vi "Main.vi"() -> ()   [LabVIEW 2018]
doc: "This template is for the Queued Message Handler design pattern.\n\nThe Event Handling Loop generates messages based on user interface actions.\n\nThe Message Handling Loop processes messages generated by the Event Handling Loop, or by other messages. The messages are string values, so new messages can be added easily to the Message Cases case structure in the Message Handling Loop. Each message cluster can also provide an optional value for Message Data, which is a variant that can be converted to whatever message-specific data is required."
uses:
  Type Defs/SR Cluster.ctl
  Type Defs/SR Status.ctl
  Type Defs/Filter Cluster.ctl
  Type Defs/Sorting Methods.ctl
  Support/Message Queue/Enqueue Message (Single).vi
  Support/Message Queue/Message Queue.lvlib
  Support/User Events/User Events.lvlib
panel:
  in  "Remove SR":bool
  in  "Legend":cluster{"Color Box":u32, "String":string}[][](array[cluster])=[[{"Color Box"=16750899, "String"="In Work (Answer Today)"}, {"Color Box"=6737151, "String"="In Collab"}, {"Color Box"=16735833, "String"="Past Due"}], [{"Color Box"=14417800, "String"="In Work"}, {"Color Box"=4713287, "String"="Potentially Resolved"}, {"Color Box"=16580608, "String"="Passed Off"}], [{"Color Box"=3342591, "String"="In Collab (Answer Today)"}, {"Color Box"=9746580, "String"="Resolved"}, {"Color Box"=0, "String"="Other"}]]
  out "Message":string
  out "Labels":string="          SR#          SR Status                          Name                                 Summary                                                                         Last Updated      SR Type                 Service Level        Open      Create Date"
  in  "Sorting":T1
  in  "Filter Cluster":T2={"Show Resolved"=TRUE, "Show Potentially Resolved"=TRUE, "Show Passoffs"=TRUE, "Show In Collab"=TRUE}
  in  "Add SR":bool
  out "SR Display List":T3[](array[typedef]) {"Creation Date" format="%<%x>T"; "Last Updated" format="%<%x>T"; "Days Open" format="%#.1f"}
  in  "Refresh SRs":bool
  in  "Exit":bool
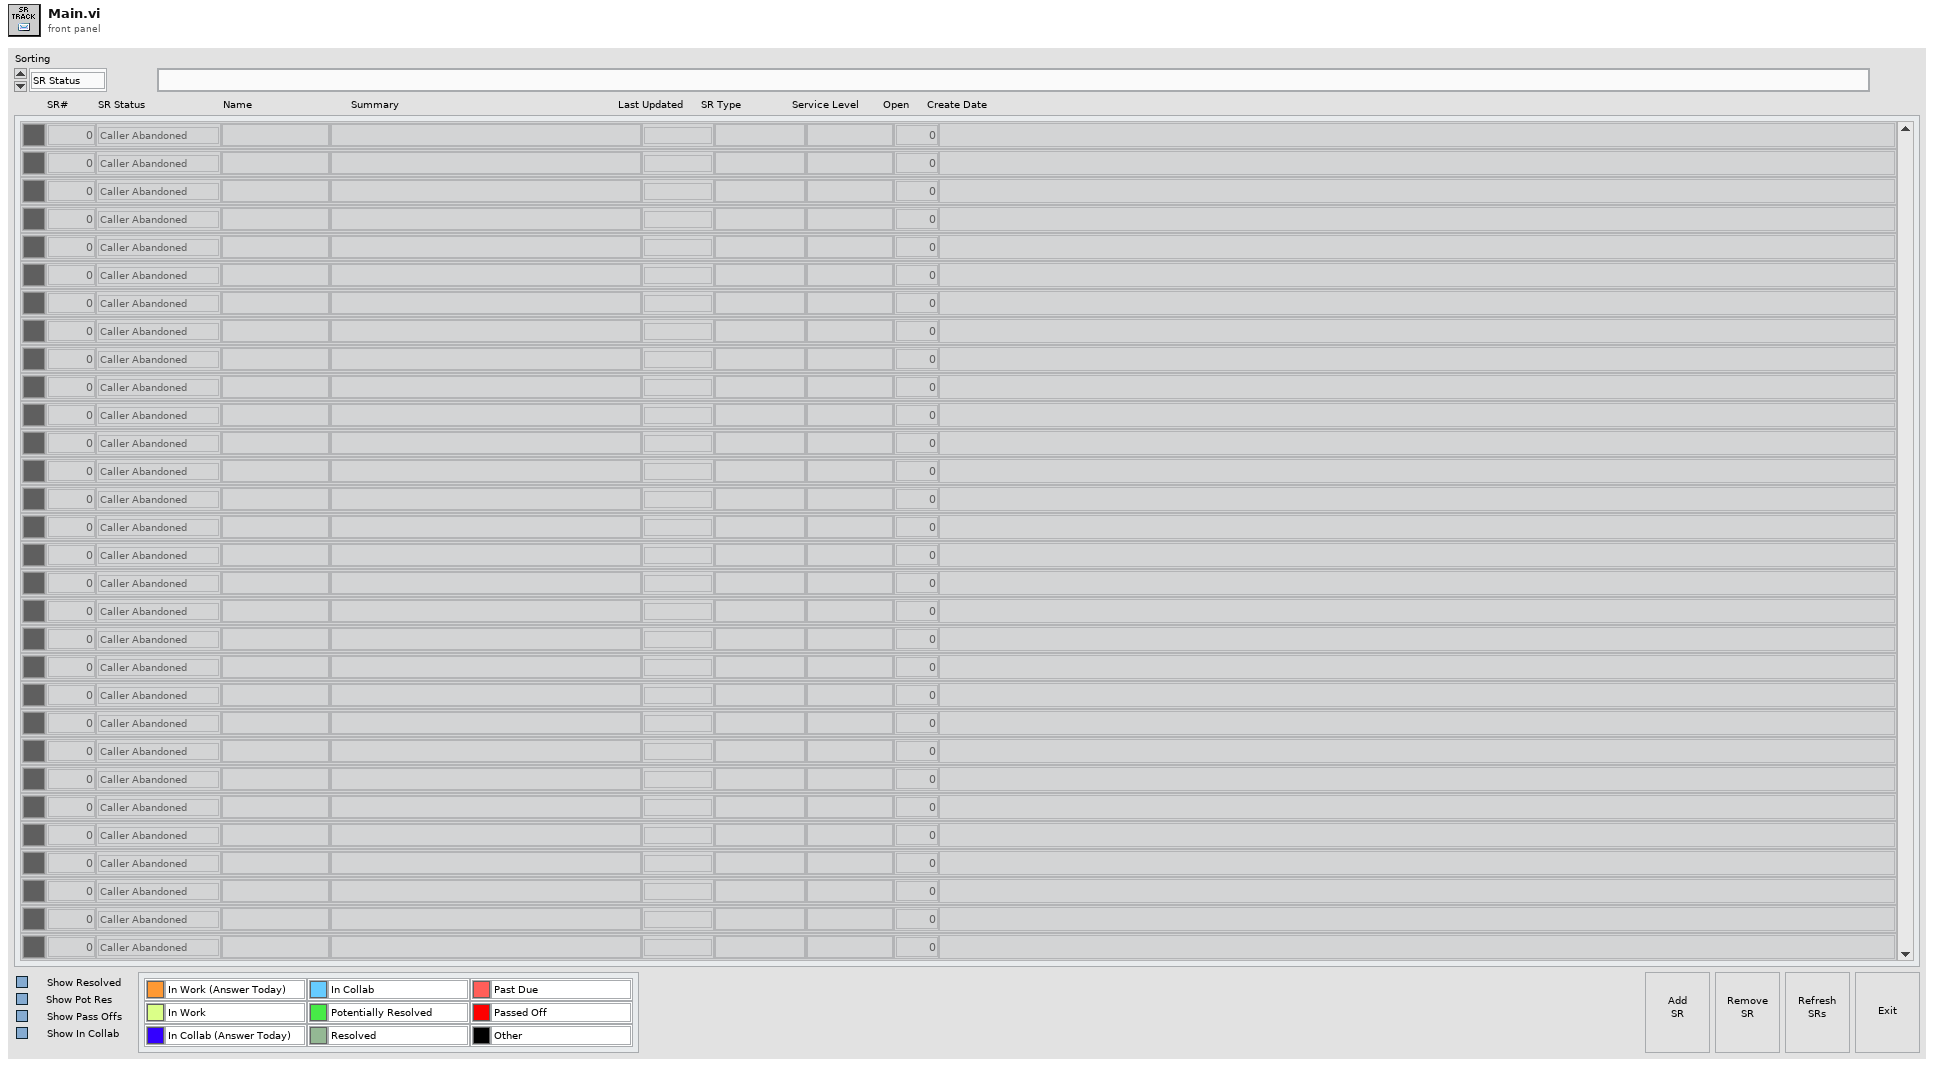
[diagram p1: front panel]
types:
  T1 = typedef "Sorting Methods.ctl" = enum16{"SR Status", "Most Recent", "SR Type", "SR Number", "Days Open", "Urgency"}
  T2 = typedef "Filter Cluster.ctl" = cluster{"Show Resolved":bool, "Show Potentially Resolved":bool, "Show Passoffs":bool, "Show In Collab":bool}
  T3 = typedef "SR Cluster.ctl" = cluster{"Color":u32, "SR Number":i32, "SR Status":T4, "Name":string, "Summary":string, "Last Updated":timestamp, "SR Type":string, "Service Level":string, "Days Open":dbl, "Creation Date":timestamp, "Owner":string, "Note":string}
  T4 = typedef "SR Status.ctl" = enum16{"Caller Abandoned", "Created in Error", "Expired", "Forum Resolved AE", "Forum Resolved Customer", "IN WORK", "IN WORK Collab with AES", "IN WORK Collab with PSE", "IN WORK Collab with SE", "IN WORK Customer Added Note", "IN WORK Escalation", "IN WORK Wait on Customer", "Open", "Potentially Resolved", "Presumed Resolved", "RMA Approved for Return", "RMA Closed", "RMA Closed - DOA", "RMA In Progress", "RMA Open", "RMA Waiting on Customer", "Resolved", "Passed Off"}
  T5 = typedef "User Events.ctl" = cluster{"Refresh":refnum<user-event>, "Stop":refnum<user-event>}
  T6 = typedef "Message Queue.lvlib/All Message Queues.ctl" = cluster{"UI":refnum<queue>, "Pop":refnum<queue>, "FileIO":refnum<queue>}
  T7 = typedef "LVPoint32TypeDef.ctl" = cluster{"Horizontal":i32, "Vertical":i32}
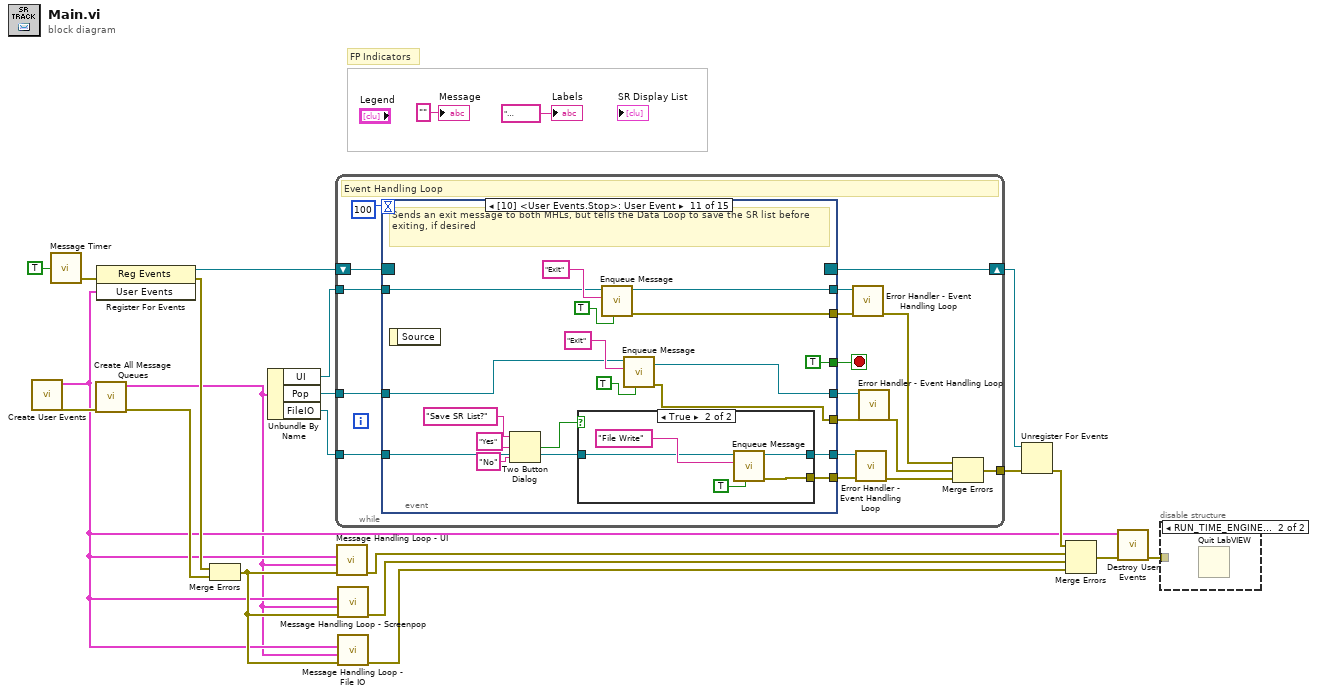
[diagram p0: block diagram]
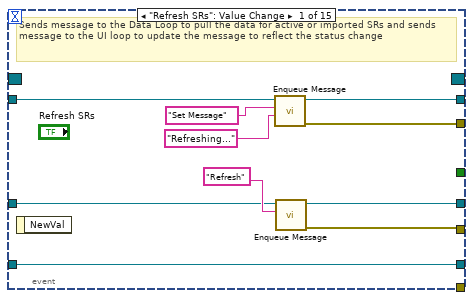
[diagram p2: hidden frame]
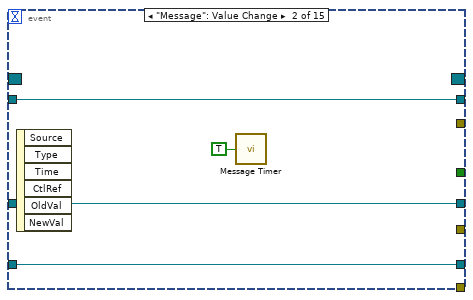
[diagram p3: hidden frame]
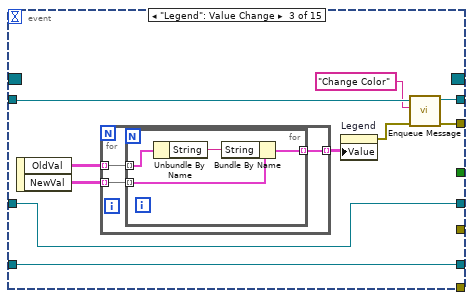
[diagram p4: hidden frame]
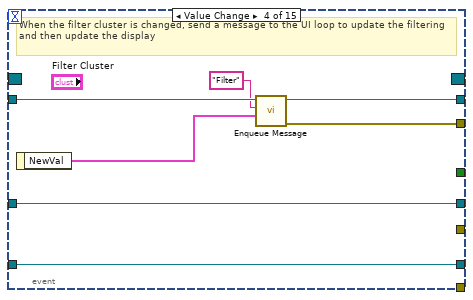
[diagram p5: hidden frame]
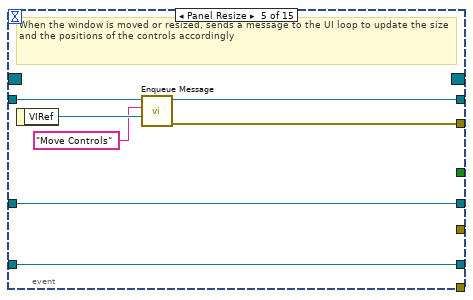
[diagram p6: hidden frame]
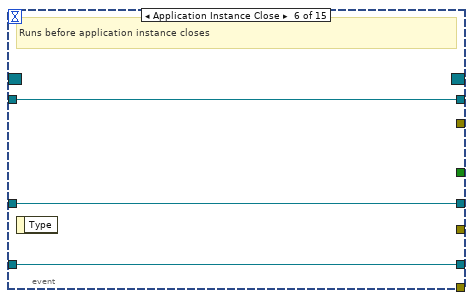
[diagram p7: hidden frame]
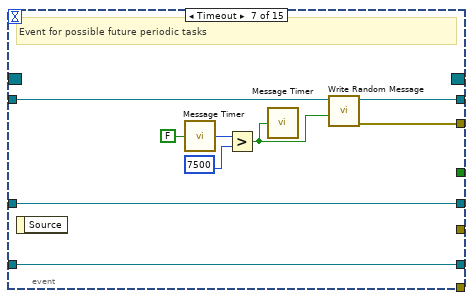
[diagram p8: hidden frame]
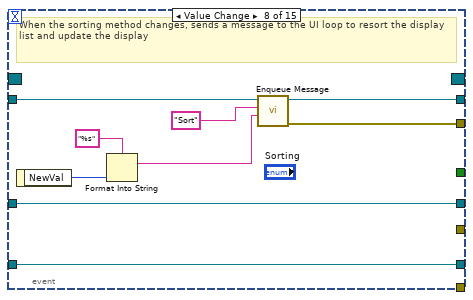
[diagram p9: hidden frame]
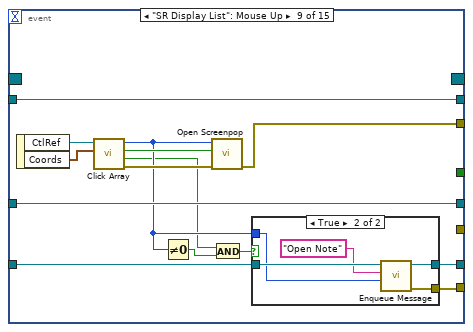
[diagram p10: hidden frame]
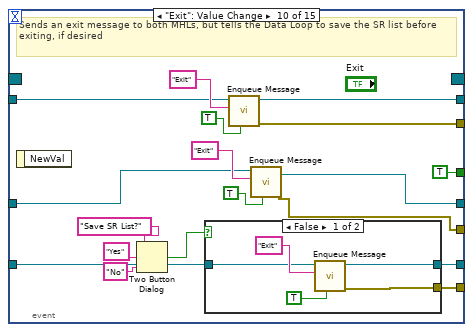
[diagram p12: hidden frame]
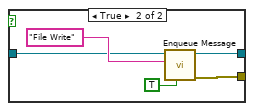
[diagram p13: hidden frame]
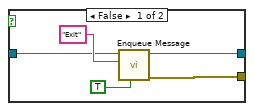
[diagram p14: hidden frame]
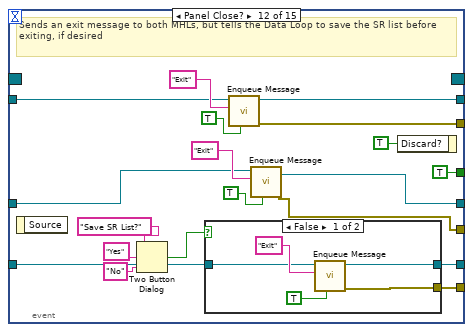
[diagram p15: hidden frame]
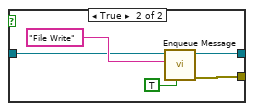
[diagram p16: hidden frame]
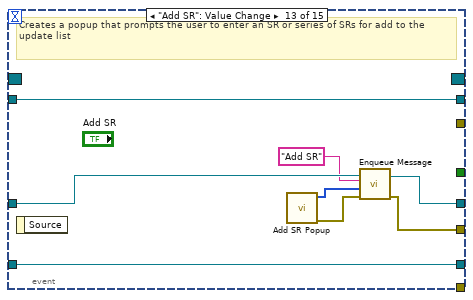
[diagram p17: hidden frame]
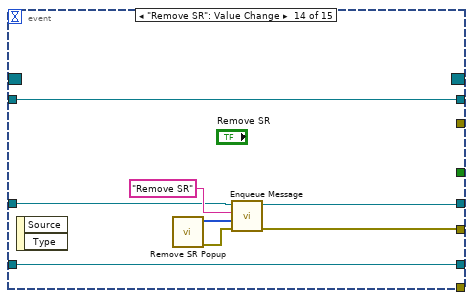
[diagram p18: hidden frame]
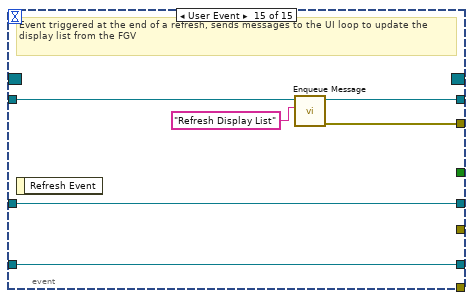
[diagram p19: hidden frame]
diagram:
  # "FP Indicators"
  n1 = call "Create User Events.vi"() -> ("error out"=w16:errorcluster, "User Events"=w3:T5)  [unwired: 10 in]
  n2 = call "Message Timer.vi"("Reset?"=TRUE) -> ("Error Out"=w6:errorcluster)  [unwired: 3 in, 1 out]
  n3 = call "Create All Message Queues.vi"("error in (no error)"=w16) -> ("error out"=w22:errorcluster, "Message Queues out"=w2:T6)  [unwired: 9 in]
  n4 = register-events(error in=w6, w3) -> (reference out=w19:refnum<event-registration>, error out=w18:errorcluster)  [unwired: 1 in]
  n5 = Merge Errors(w18, w22) -> (w4:errorcluster)
  n6 = Unbundle By Name(w2) -> ("UI"=w8:refnum<queue>, "Pop"=w9:refnum<queue>, "FileIO"=w5:refnum<queue>)
  n7 = while {
    tunnel: w8 -> [w39]
    shift-right: [w37] -> w20
    shift-left: w19 -> [w38]
    tunnel: [w32] -> w17
    tunnel: w9 -> [w31]
    tunnel: w5 -> [w24]
    stop <- w35 stop-if-true
    # "Event Handling Loop"
    n8 = event shown="[10] <User Events.Stop>: User Event" {
      selector: w38 -> [_ _ _ _ _ _ _ _ _ _ _ _ _ _ _]
      dyn-events: [_ _ _ _ _ _ _ _ _ _ _ _ _ _ _] -> w37
      timeout: 100 -> [_ _ _ _ _ _ _ _ _ _ _ _ _ _ _]
      tunnel: [_ _ _ _ _ _ _ _ _ TRUE ("Discard?") TRUE ("Discard?") TRUE ("Discard?") _ _ _] -> w35
      tunnel: w39 -> [w43 w53 w56 w76 w83 w86 w93 w102 w119 w135 w164 w192 w218 w226 w231]
      tunnel: [w41 _ w58 w74 w81 _ w90 w103 w114 w137 w166 w194 _ _ w227] -> w36
      tunnel: [w46 w53 w59 w75 w82 w86 w94 w104 w119 w136 w165 w193 w218 w226 w230] -> w34
      tunnel: [w49 w52 w61 w77 w84 w87 w92 w105 w118 w129 w158 w186 w215 w223 w232] -> w33
      tunnel: w31 -> [w42 w52 w61 w77 w84 w87 w92 w105 w118 w126 w156 w183 w217 w224 w232]
      tunnel: [w47 _ _ _ _ _ _ _ _ w127 w154 w184 w212 w222 _] -> w29
      tunnel: [w40 w50 w54 w71 w78 w85 w88 w97 w113 w134 w163 w191 w213 w219 w228] -> w25
      tunnel: w24 -> [w40 w50 w54 w71 w78 w85 w88 w97 w111 w132 w161 w189 w213 w219 w228]
      tunnel: [_ _ _ _ _ _ _ _ w112 w133 w162 w190 _ _ _] -> w23
      event "Refresh SRs": Value Change {
        # "Sends message to the Data Loop to pull the data for active or imported SRs and sends message to the UI loop to update the message to reflect the status change"
        n9 = event-data() -> ()  [unwired: 1 in, 1 out]
        n10 = call-poly "Enqueue Message.vi"("Message Data"="Refreshing..." ("Message"), "Message"="Set Message", "Message Queue"=w43) -> ("error out"=w41:errorcluster, "dup Message Queue"=w46:refnum<queue>)  [unwired: 7 in]
        n11 = call-poly "Enqueue Message.vi"("Message"="Refresh", "Message Queue"=w42) -> ("error out"=w47:errorcluster, "dup Message Queue"=w49:refnum<queue>)  [unwired: 8 in]
      }
      event "Message": Value Change {
        n12 = event-data() -> ()  [unwired: 1 in, 6 out]
        n13 = call "Message Timer.vi"("Reset?"=TRUE) -> ()  [unwired: 3 in, 2 out]
      }
      event "Legend": Value Change {
        n14 = event-data() -> ("OldVal"=w62:cluster{"Color Box":u32, "String":string}[][], "NewVal"=w63:cluster{"Color Box":u32, "String":string}[][])  [unwired: 1 in]
        n15 = for {
          tunnel: w63 -> [w66] mode=indexing
          tunnel: w62 -> [w65] mode=indexing
          tunnel: [w64] -> w60 mode=indexing
          n16 = for {
            tunnel: w66 -> [w67] mode=indexing
            tunnel: w65 -> [w70] mode=indexing
            tunnel: [w68] -> w64 mode=indexing
            n17 = Unbundle By Name(w70) -> ("String"=w69:string)
            n18 = Bundle By Name(cluster=w67, "String"=w69) -> (w68:cluster{"Color Box":u32, "String":string})
          }
        }
        n19 = property on="Legend" class="Arr (strict)"("Value"=w60) -> (error out=w57:errorcluster)  [unwired: 2 in, 1 out]
        n20 = call-poly "Enqueue Message.vi"("error in (no error)"=w57, "Message"="Change Color", "Message Queue"=w56) -> ("error out"=w58:errorcluster, "dup Message Queue"=w59:refnum<queue>)  [unwired: 7 in]
      }
      event Value Change {
        # "When the filter cluster is changed, send a message to the UI loop to update the filtering and then update the display"
        n21 = event-data() -> ("NewVal"=w72:T2)  [unwired: 1 in]
        n22 = call-poly "Enqueue Message.vi"("Message Data"=w72, "Message"="Filter", "Message Queue"=w76) -> ("error out"=w74:errorcluster, "dup Message Queue"=w75:refnum<queue>)  [unwired: 7 in]
      }
      event Panel Resize {
        # "When the window is moved or resized, sends a message to the UI loop to update the size and the positions of the controls accordingly"
        n23 = event-data() -> ("VIRef"=w80:refnum<vi>)  [unwired: 1 in]
        n24 = call-poly "Enqueue Message.vi"("Message Data"=w80, "Message"="Move Controls", "Message Queue"=w83) -> ("error out"=w81:errorcluster, "dup Message Queue"=w82:refnum<queue>)  [unwired: 7 in]
      }
      event Application Instance Close {
        # "Runs before application instance closes"
        n25 = event-data() -> ()  [unwired: 1 in, 1 out]
      }
      event Timeout {
        # "Event for possible future periodic tasks"
        n26 = event-data() -> ()  [unwired: 1 in, 1 out]
        n27 = call "Message Timer.vi"("Reset?"=FALSE) -> ("Timer Count"=w96:u32)  [unwired: 3 in, 1 out]
        n28 = Greater?(x=w96, y=u32 7500) -> (0:w89:bool)
        n29 = call "Message Timer.vi"("Reset?"=w89) -> ()  [unwired: 3 in, 2 out]
        n30 = call "Write Random Message.vi"("Send Message?"=w89, "Queue in"=w93) -> ("error out"=w90:errorcluster, "Queue out"=w94:refnum<queue>)  [unwired: 8 in]
      }
      event Value Change {
        # "When the sorting method changes, sends a message to the UI loop to resort the display list and update the display"
        n31 = event-data() -> ("NewVal"=w100:T1)  [unwired: 1 in]
        n32 = Format Into String(format string="%s", w100) -> (resulting string=w98:string)  [unwired: 2 in, 1 out]
        n33 = call-poly "Enqueue Message.vi"("Message Data"=w98, "Message"="Sort", "Message Queue"=w102) -> ("error out"=w103:errorcluster, "dup Message Queue"=w104:refnum<queue>)  [unwired: 7 in]
      }
      event "SR Display List": Mouse Up {
        n34 = event-data() -> ("CtlRef"=w115:refnum<vi>, "Coords"=w117:T7)  [unwired: 1 in]
        n35 = call "Click Array.vi"("Coords"=w117, "CtlRef"=w115) -> ("error out"=w116:errorcluster, "Open Note?"=w106:bool, "Open Screenpop?"=w109:bool, "SR Number"=w107:i32)  [unwired: 6 in]
        n36 = Not Equal To 0?(x=w107) -> (x != 0?=w108:bool)
        n37 = call "Open Screenpop.vi"("error in (no error)"=w116, "Open?"=w109, "SR Number"=w107) -> ("error out"=w114:errorcluster)  [unwired: 8 in]
        n38 = And(x=w106, y=w108) -> (x .and. y?=w110:bool)
        n39 = case shown="True" w110 {
          tunnel: [w120 w125] -> w113
          tunnel: [_ w124] -> w112
          tunnel: w111 -> [w120 w123]
          tunnel: w107 -> [_ w121]
          frame False {
          }
          frame True {
            n40 = call-poly "Enqueue Message.vi"("Message Data"=w121, "Message"="Open Note", "Message Queue"=w123) -> ("error out"=w124:errorcluster, "dup Message Queue"=w125:refnum<queue>)  [unwired: 7 in]
          }
        }
      }
      event "Exit": Value Change {
        # "Sends an exit message to both MHLs, but tells the Data Loop to save the SR list before exiting, if desired"
        n41 = event-data() -> ()  [unwired: 1 in, 1 out]
        n42 = Two Button Dialog(message="Save SR List?", 1:"No" ("F button name (\"Cancel\")"), 2:"Yes" ("T button name (\"OK\")")) -> (T button?=w138:bool)
        n43 = case shown="False" w138 {
          tunnel: [w145 w152] -> w133
          tunnel: [w146 w151] -> w134
          tunnel: w132 -> [w147 w149]
          frame False {
            n44 = call-poly "Enqueue Message.vi"("Priority Message? (F)"=TRUE, "Message"="Exit", "Message Queue"=w147) -> ("error out"=w145:errorcluster, "dup Message Queue"=w146:refnum<queue>)  [unwired: 7 in]
          }
          frame True {
            n45 = call-poly "Enqueue Message.vi"("Priority Message? (F)"=TRUE, "Message"="File Write", "Message Queue"=w149) -> ("error out"=w152:errorcluster, "dup Message Queue"=w151:refnum<queue>)  [unwired: 7 in]
          }
        }
        n46 = call-poly "Enqueue Message.vi"("Priority Message? (F)"=TRUE, "Message"="Exit", "Message Queue"=w135) -> ("error out"=w137:errorcluster, "dup Message Queue"=w136:refnum<queue>)  [unwired: 7 in]
        n47 = call-poly "Enqueue Message.vi"("Priority Message? (F)"=TRUE, "Message"="Exit", "Message Queue"=w126) -> ("error out"=w127:errorcluster, "dup Message Queue"=w129:refnum<queue>)  [unwired: 7 in]
      }
      event User Event {
        # "Sends an exit message to both MHLs, but tells the Data Loop to save the SR list before exiting, if desired"
        n48 = event-data() -> ()  [unwired: 1 in, 1 out]
        n49 = Two Button Dialog(message="Save SR List?", 1:"No" ("F button name (\"Cancel\")"), 2:"Yes" ("T button name (\"OK\")")) -> (T button?=w167:bool)
        n50 = case shown="True" w167 {
          tunnel: [w173 w180] -> w162
          tunnel: [w174 w179] -> w163
          tunnel: w161 -> [w175 w177]
          frame False {
            n51 = call-poly "Enqueue Message.vi"("Priority Message? (F)"=TRUE, "Message"="Exit", "Message Queue"=w175) -> ("error out"=w173:errorcluster, "dup Message Queue"=w174:refnum<queue>)  [unwired: 7 in]
          }
          frame True {
            n52 = call-poly "Enqueue Message.vi"("Priority Message? (F)"=TRUE, "Message"="File Write", "Message Queue"=w177) -> ("error out"=w180:errorcluster, "dup Message Queue"=w179:refnum<queue>)  [unwired: 7 in]
          }
        }
        n53 = call-poly "Enqueue Message.vi"("Priority Message? (F)"=TRUE, "Message"="Exit", "Message Queue"=w164) -> ("error out"=w166:errorcluster, "dup Message Queue"=w165:refnum<queue>)  [unwired: 7 in]
        n54 = call-poly "Enqueue Message.vi"("Priority Message? (F)"=TRUE, "Message"="Exit", "Message Queue"=w156) -> ("error out"=w154:errorcluster, "dup Message Queue"=w158:refnum<queue>)  [unwired: 7 in]
      }
      event Panel Close? {
        # "Sends an exit message to both MHLs, but tells the Data Loop to save the SR list before exiting, if desired"
        n55 = event-data() -> ()  [unwired: 1 in, 1 out]
        n56 = Two Button Dialog(message="Save SR List?", 1:"No" ("F button name (\"Cancel\")"), 2:"Yes" ("T button name (\"OK\")")) -> (T button?=w195:bool)
        n57 = case shown="False" w195 {
          tunnel: [w202 w209] -> w190
          tunnel: [w203 w208] -> w191
          tunnel: w189 -> [w204 w206]
          frame False {
            n58 = call-poly "Enqueue Message.vi"("Priority Message? (F)"=TRUE, "Message"="Exit", "Message Queue"=w204) -> ("error out"=w202:errorcluster, "dup Message Queue"=w203:refnum<queue>)  [unwired: 7 in]
          }
          frame True {
            n59 = call-poly "Enqueue Message.vi"("Priority Message? (F)"=TRUE, "Message"="File Write", "Message Queue"=w206) -> ("error out"=w209:errorcluster, "dup Message Queue"=w208:refnum<queue>)  [unwired: 7 in]
          }
        }
        n60 = call-poly "Enqueue Message.vi"("Priority Message? (F)"=TRUE, "Message"="Exit", "Message Queue"=w192) -> ("error out"=w194:errorcluster, "dup Message Queue"=w193:refnum<queue>)  [unwired: 7 in]
        n61 = call-poly "Enqueue Message.vi"("Priority Message? (F)"=TRUE, "Message"="Exit", "Message Queue"=w183) -> ("error out"=w184:errorcluster, "dup Message Queue"=w186:refnum<queue>)  [unwired: 7 in]
        n62 = event-data("Discard?"=TRUE) -> ()  [unwired: 1 in, 1 out]
      }
      event "Add SR": Value Change {
        # "Creates a popup that prompts the user to enter an SR or series of SRs for add to the update list"
        n63 = event-data() -> ()  [unwired: 1 in, 1 out]
        n64 = call "Add SR Popup.vi"() -> ("error out"=w216:errorcluster, "SR array out"=w211:i32[])  [unwired: 9 in, 1 out]
        n65 = call-poly "Enqueue Message.vi"("error in (no error)"=w216, "Message Data"=w211, "Message"="Add SR", "Message Queue"=w217) -> ("error out"=w212:errorcluster, "dup Message Queue"=w215:refnum<queue>)  [unwired: 6 in]
      }
      event "Remove SR": Value Change {
        n66 = event-data() -> ()  [unwired: 1 in, 2 out]
        n67 = call "Remove SR Popup.vi"() -> ("error out"=w220:errorcluster, "SR array out"=w221:i32[])  [unwired: 10 in]
        n68 = call-poly "Enqueue Message.vi"("error in (no error)"=w220, "Message Data"=w221, "Message"="Remove SR", "Message Queue"=w224) -> ("error out"=w222:errorcluster, "dup Message Queue"=w223:refnum<queue>)  [unwired: 6 in]
      }
      event User Event {
        # "Event triggered at the end of a refresh, sends messages to the UI loop to update the display list from the FGV"
        n69 = event-data() -> ()  [unwired: 1 in, 1 out]
        n70 = call-poly "Enqueue Message.vi"("Message"="Refresh Display List", "Message Queue"=w231) -> ("error out"=w227:errorcluster, "dup Message Queue"=w230:refnum<queue>)  [unwired: 8 in]
      }
    }
    n71 = call "Error Handler - Event Handling Loop.vi"("error in (no error)"=w36, "Message Queue"=w34) -> ("dup error in"=w27:errorcluster)  [unwired: 8 in, 1 out]
    n72 = call "Error Handler - Event Handling Loop.vi"("error in (no error)"=w23, "Message Queue"=w25) -> ("dup error in"=w26:errorcluster)  [unwired: 8 in, 1 out]
    n73 = call "Error Handler - Event Handling Loop.vi"("error in (no error)"=w29, "Message Queue"=w33) -> ("dup error in"=w28:errorcluster)  [unwired: 8 in, 1 out]
    n74 = Merge Errors(w27, w28, w26) -> (w32:errorcluster)
  }
  n75 = call "Message Handling Loop - UI.vi"("error in"=w4, "Message Queues in"=w2, "User Event Bundle"=w3) -> ("error out"=w10:errorcluster)  [unwired: 8 in]
  n76 = call "Message Handling Loop - Screenpop.vi"("error in"=w4, "Message Queues in"=w2, "User Event Bundle"=w3) -> ("error out"=w11:errorcluster)  [unwired: 8 in]
  n77 = call "Message Handling Loop - File IO.vi"("error in"=w4, "Message Queues in"=w2, "User Event Bundle"=w3) -> ("error out"=w1:errorcluster)  [unwired: 8 in]
  n78 = Unregister For Events(event registration refnum=w20, error in=w17) -> (error out=w21:errorcluster)
  n79 = Merge Errors(w21, w10, w11, w1) -> (w15:errorcluster)
  n80 = call "Destroy User Events.vi"("error in (no error)"=w15, "User Event Bundle"=w3) -> ("error out"=w14:errorcluster)  [unwired: 9 in]
  n81 = disable-structure shown="RUN_TIME_ENGINE==True" {
    disable-tunnel: w14 -> [_ _]
    frame condition #0 (active) {
    }
    frame condition #1 {
      n82 = Quit LabVIEW() -> ()  [unwired: 1 in]
    }
  }
  "Message" <- "" ("Message")
  "Labels" <- "           SR#          SR Status                          Name                         Summary                                                                                        Updated        SR Type                 Service Level        Open   Note" ("Labels")
